vi "INIT.vi"(8 "error in (no error)":errorcluster, 11 "DLOwis in":refnum<class "DLOwis.lvclass">) -> (0 "error out":errorcluster, 3 "DLOwis out":refnum<class "DLOwis.lvclass">)   [LabVIEW 2018, in "DLOwis.lvclass"]
uses:
  DLOwis.lvclass
  C:/Users/Sergey Denisov/Documents/REPS/TRANCON/Classes/GeneralFunctionality/GeneralFunctionality.lvclass
  GeneralFunctionality/GeneralFunctionality.lvclass/GeneralFunctionality.ctl
  dependecies/ControlsVIs/Clusters-def/SERVER-Commands.ctl
  dependecies/ControlsVIs/Clusters-def/Message types.ctl
  Control/Control-Server/Control-Server.lvclass
  Message/Message.lvclass
  GeneralFunctionality/GeneralFunctionality.lvclass
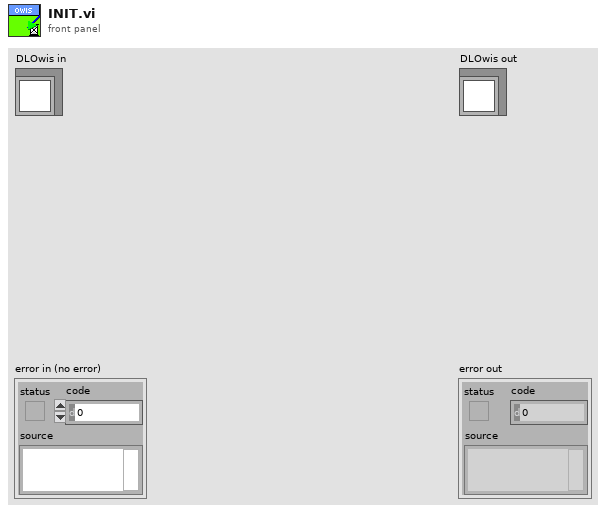
[diagram p1: front panel]
types:
  T1 = typedef "Message types.ctl" = string
  T2 = typedef "Control-Server.lvclass/SERVER-Commands.ctl" = string
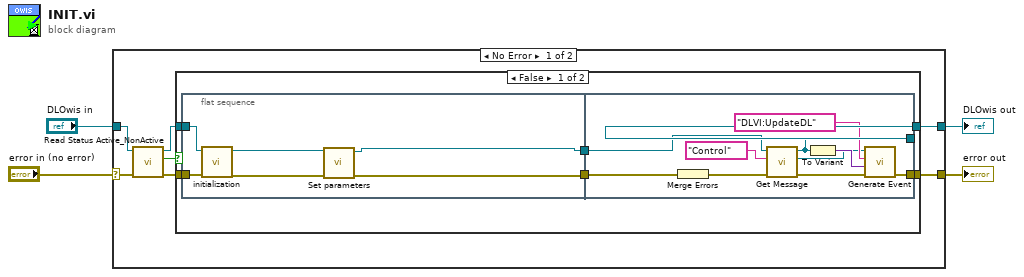
[diagram p0: block diagram]
diagram:
  n1 = case shown="No Error" "error in (no error)" {
    selector: "error in (no error)" -> [w8 w36]
    tunnel: "DLOwis in" -> [w9 w37]
    tunnel: [w11 w37] -> w4
    tunnel: [w10 w36] -> w3
    frame No Error {
      n2 = call "Read Status Active_NonActive.vi"("error in (no error)"=w8, "GeneralFunctionality in"=w9) -> ("error out"=w5:errorcluster, "Status Active/NonActive"=w7:bool, "GeneralFunctionality out"=w6:refnum<class "DLOwis.lvclass">)  [unwired: 7 in]
      n3 = case shown="False" w7 {
        tunnel: [w13 w35] -> w11
        tunnel: [w15 w34] -> w10
        tunnel: w6 -> [w17 w35]
        tunnel: w5 -> [w16 w34]
        frame False {
          n4 = flat-sequence {
            tunnel: w17 -> [w23]
            tunnel: w16 -> [w22]
            tunnel: [w20] -> w14
            tunnel: [w19] -> w12
            tunnel: w14 -> [w28]
            tunnel: [w30] -> w15
            tunnel: [w27] -> w13
            tunnel: w12 -> [w25]
            frame #0 {
              n5 = call "initialization.vi"("error in (no error)"=w22, "DLOwis in"=w23) -> ("error out"=w18:errorcluster, "DLOwis out"=w21:refnum<class "DLOwis.lvclass">)  [unwired: 8 in]
              n6 = call-dynamic "Set parameters.vi"("error in (no error)"=w18, "DLOwis en entrée"=w21) -> ("error out"=w19:errorcluster, "DLOwis en sortie"=w20:refnum<class "DLOwis.lvclass">)  [unwired: 8 in]
            }
            frame #1 {
              n7 = Merge Errors(w25) -> (w24:errorcluster)
              n8 = call "Get Message.vi"("error in (no error)"=w24, "Message type"=T1 "Control", "GeneralFunctionality en entrée"=w28) -> ("error out"=w31:errorcluster, "Message.lvclass"=w29:refnum<class "Message.lvclass">, "GeneralFunctionality en sortie"=w27:refnum<class "DLOwis.lvclass">)  [unwired: 6 in]
              n9 = To Variant(anything=w27) -> (Variant=w33:variant)
              n10 = call "Generate Event.vi"("error in (no error)"=w31, "Data"=w33, "Command"=T2 "DLVI:UpdateDL", "Message en entrée"=w29) -> ("error out"=w30:errorcluster)  [unwired: 6 in, 1 out]
            }
          }
        }
        frame True {
        }
      }
    }
    frame Error {
    }
  }
  "error out" <- w3
  "DLOwis out" <- w4
